vi "Aula02.vi"() -> ()   [LabVIEW 2024]
panel:
  out "s? t:f":dbl[](array[numeric])
  in  "Boolean 2":bool
  out "Boolean":bool
  out "String":string
  in  "N Value":dbl
  out "Slide":dbl(slide) scale=0.0..200.0
  in  "Array 2 - 1":dbl
  in  "Array 2 - 0":dbl
  out "I value":i32
  in  "Array 1 -1":dbl
  in  "Array 1 - 0":dbl
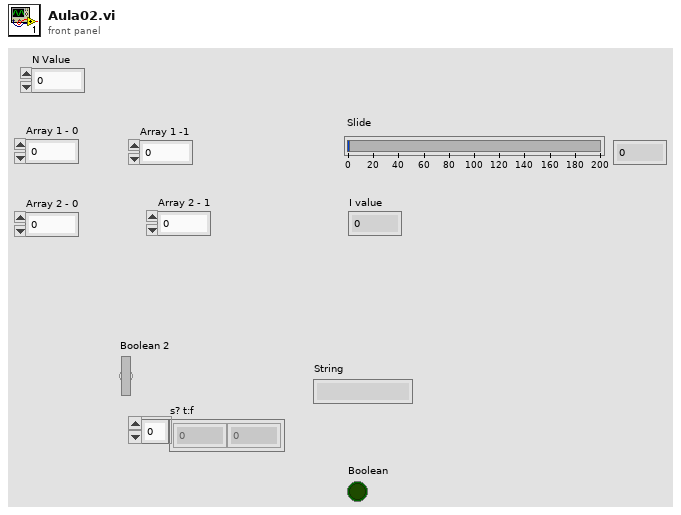
[diagram p1: front panel]
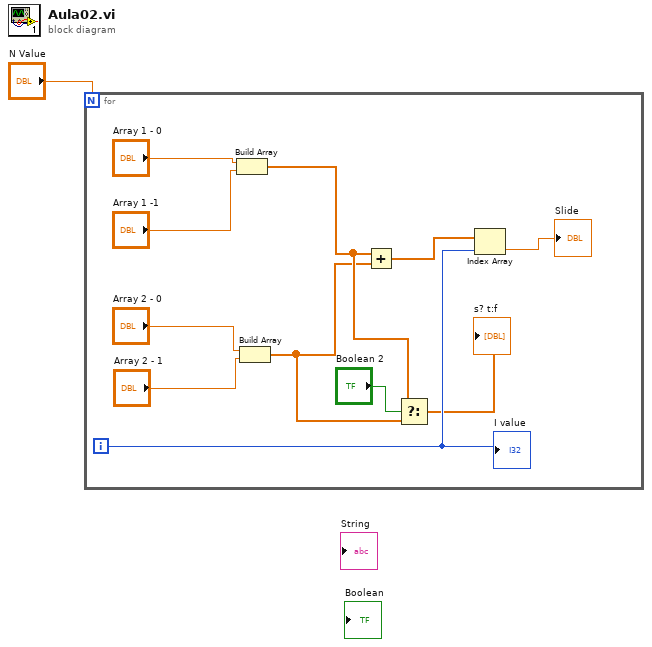
[diagram p0: block diagram]
diagram:
  n1 = for {
    N: "N Value" -> [_]
    i -> [w7]
    n2 = Build Array("Array 1 - 0", "Array 1 -1") -> (w5:dbl[])
    n3 = Build Array("Array 2 - 0", "Array 2 - 1") -> (w4:dbl[])
    n4 = Add(x=w5, y=w4) -> (x+y=w8:dbl[])
    n5 = Select(t=w5, s="Boolean 2", f=w4) -> (s? t:f=→"s? t:f":dbl[])
    n6 = Index Array(array=w8, index=w7) -> (element=→"Slide":dbl)
    "I value" <- w7
  }
